vi "Ball.vi"() -> ()   [LabVIEW 2015]
uses:
  <vilib>/LabVIEW Interface for Arduino/Type Defs/Board Type.ctl
  <vilib>/LabVIEW Interface for Arduino/LabVIEW Interface for Arduino.lvlib
  <vilib>/ptbypt/NI_PtbyPt.lvlib
panel:
  out "Waveform Chart 6":dbl(graph)
  in  "Slide":dbl(slide) scale=-20.0..20.0
  out "Waveform Chart 5":dbl(graph)
  in  "Kd":dbl=4.05
  in  "Kp":dbl=0.3 format="%#_13g"
  out "Waveform Chart 4":dbl(graph)
  out "Waveform Chart 3":dbl(graph)
  out "Waveform Chart 2":dbl(graph)
  out "Waveform Chart":dbl(graph)
  in  "stop":bool
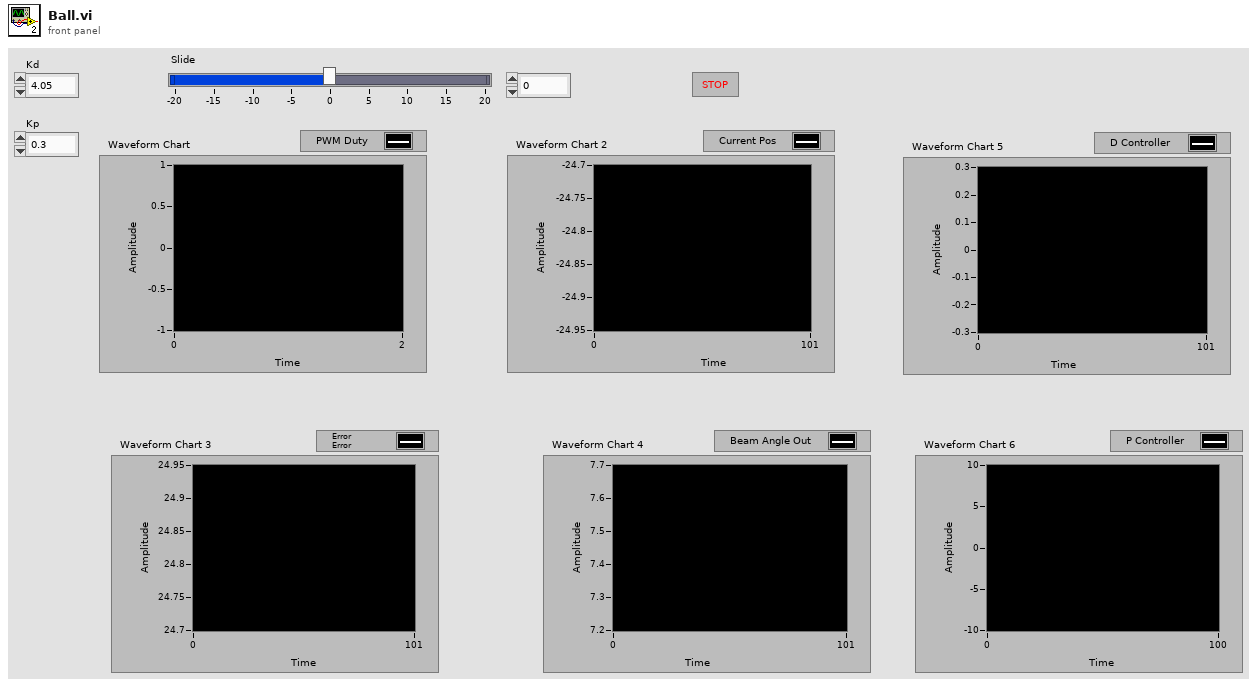
[diagram p1: front panel]
types:
  T1 = typedef "LabVIEW Interface for Arduino.lvlib/Board Type.ctl" = enum16{"Uno", "Dimuelanove w/Atmega 328", "Mega 2560"}
  T2 = typedef "LabVIEW Interface for Arduino.lvlib/Arduino Resource.ctl" = cluster{"VISA resource":refnum<visa-resource-name>, "Board Type":T1, "Connection Type":enum8{"USB / Serial"}, "Bytes Per Packet (15)":u8}
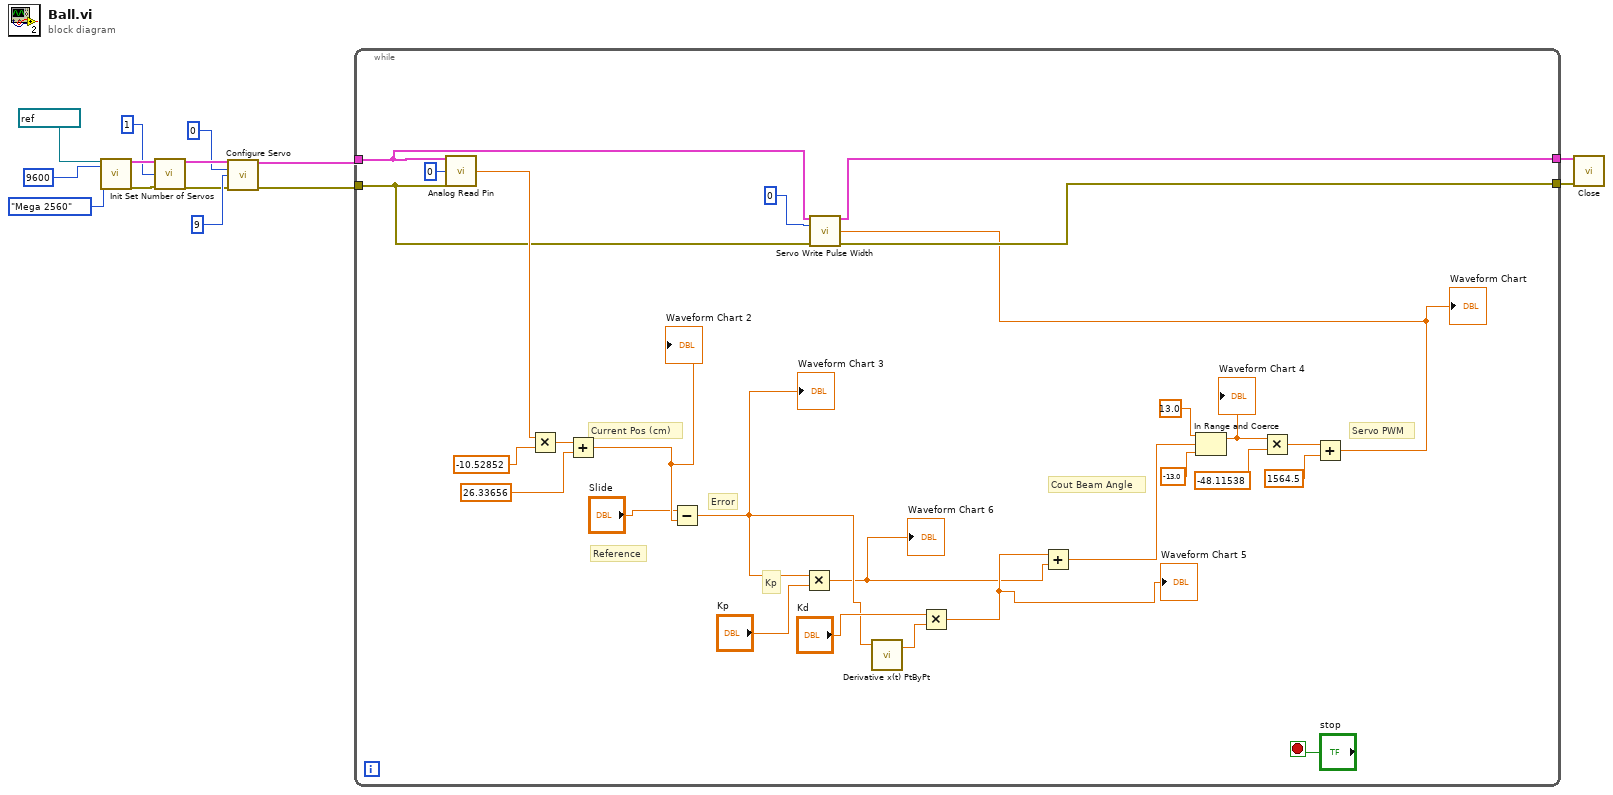
[diagram p0: block diagram]
diagram:
  n1 = call <vilib>:"Init.vi"("VISA resource"=refnum<visa-resource-name> "COM8", "Baud Rate (115200)"=u32 9600, "Board Type (Uno)"=Board_Type."Mega 2560") -> ("Arduino Resource"=w6:T2, "error out"=w5:errorcluster)  [unwired: 15 in]
  n2 = call <vilib>:"Set Number of Servos.vi"("Arduino Resource"=w6, "Number Of Servos (1)"=u8 1, "error in"=w5) -> ("Arduino Resource"=w3:T2, "error out"=w2:errorcluster)  [unwired: 11 in]
  n3 = call <vilib>:"Configure Servo.vi"("Arduino Resource"=w3, "Servo Number (0)"=u8 0, "DIO Pin (2)"=u8 9, "error in"=w2) -> ("Arduino Resource"=w9:T2, "error out"=w8:errorcluster)  [unwired: 10 in]
  n4 = while {
    tunnel: w9 -> [w29]
    tunnel: w8 -> [w22]
    tunnel: [w32] -> w11
    tunnel: [w31] -> w10
    stop <- "stop" stop-if-true
    # "Servo PWM"
    # "Cout Beam Angle"
    # "Kp"
    # "Reference"
    # "Error"
    # "Current Pos (cm)"
    n5 = call <vilib>:"Analog Read Pin.vi"("Arduino Resource"=w29, "Analog Input Pin (0)"=u8 0, "error in"=w22) -> ("Voltage"=w36:dbl)  [unwired: 10 in, 2 out]
    n6 = Multiply(x=w36, y=-10.52852) -> (x*y=w34:dbl)
    n7 = Add(x=w34, y=26.33656) -> (x+y=w25:dbl)
    "Waveform Chart 2" <- w25
    n8 = Subtract(x="Slide", y=w25) -> (x-y=w19:dbl)
    "Waveform Chart 3" <- w19
    n9 = Multiply(x=w19, y="Kp") -> (x*y=w15:dbl)
    "Waveform Chart 6" <- w15
    n10 = call <vilib>:"Derivative x(t) PtByPt.vi"("x"=w19) -> ("dx/dt"=w21:dbl)  [unwired: 3 in, 1 out]
    n11 = Multiply(x="Kd", y=w21) -> (x*y=w16:dbl)
    "Waveform Chart 5" <- w16
    n12 = Add(x=w16, y=w15) -> (x+y=w17:dbl)
    n13 = In Range and Coerce(upper limit=13.0, x=w17, lower limit=-13.0) -> (coerced(x)=w24:dbl)  [unwired: 1 out]
    "Waveform Chart 4" <- w24
    n14 = Multiply(x=w24, y=-48.11538) -> (x*y=w27:dbl)
    n15 = Add(x=w27, y=1564.5) -> (x+y=w23:dbl)
    "Waveform Chart" <- w23
    n16 = call <vilib>:"Servo Write Pulse Width.vi"("Arduino Resource"=w29, "Servo Number"=u8 0, "Pulse Width in uS"=w23, "error in"=w22) -> ("Arduino Resource"=w32:T2, "error out"=w31:errorcluster)  [unwired: 10 in]
  }
  n17 = call <vilib>:"Close.vi"("Arduino Resource"=w11, "error in"=w10) -> ()  [unwired: 13 in, 1 out]
